vi "convertVideo.vi"(8 "error in (no error)":errorcluster, 9 "format":string, 10 "fileName":string, 11 "VideoConversionFacade in":refnum<class "VideoConversionFacade.lvclass">) -> (0 "error out":errorcluster, 2 "result out":refnum<class "VideoFile.lvclass">, 3 "VideoConversionFacade out":refnum<class "VideoConversionFacade.lvclass">)   [LabVIEW 2017, in "VideoConversionFacade.lvclass"]
uses:
  VideoConversionFacade.lvclass
  VideoFile Class/VideoFile.lvclass
  CodecFactory Class/CodecFactory.lvclass
  BitrateReader Class/BitrateReader.lvclass
  AudioMixer Class/AudioMixer.lvclass
  ConsoleOut/Print Options.ctl
  OggCompressionCodec Class/OggCompressionCodec.lvclass
  C:/Users/fflores/Documents/LabVIEW-Open-Projects/LabIVEW OOP Design Patterns/Facade Pattern/Codec Class/Codec.lvclass
  MPEG4CompressionCodec Class/MPEG4CompressionCodec.lvclass
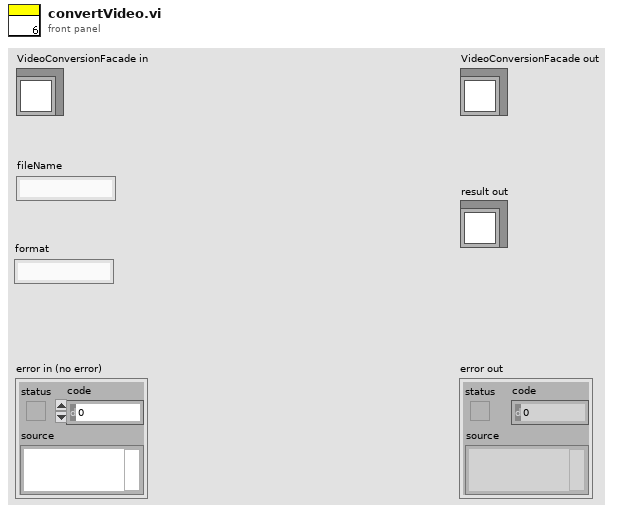
[diagram p1: front panel]
types:
  T1 = typedef "Print Options.ctl" = enum16{"Create", "Get Reference", "Print", "Print Header", "Close"}
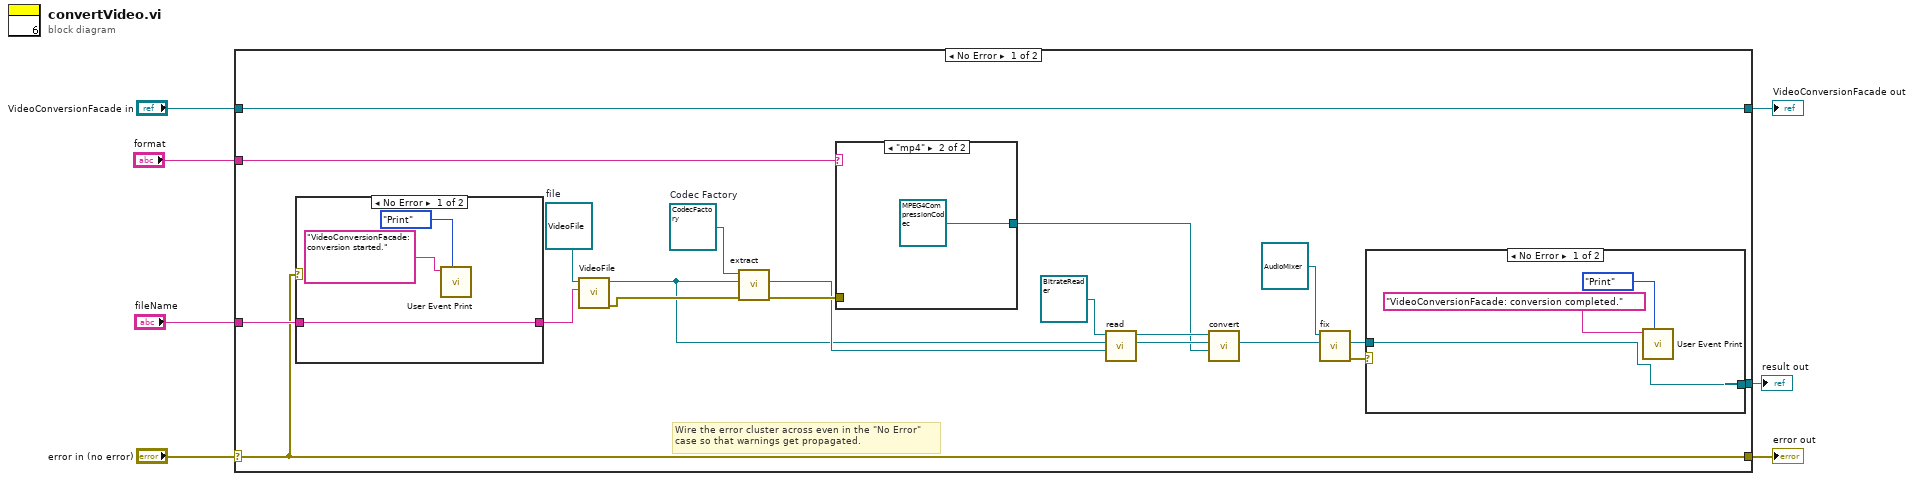
[diagram p0: block diagram]
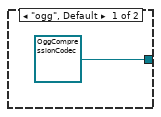
[diagram p4: hidden frame]
diagram:
  n1 = case shown="No Error" "error in (no error)" {
    selector: "error in (no error)" -> [w10 w38]
    tunnel: [w10 w38] -> w6
    tunnel: [w27 w37] -> w4
    tunnel: "VideoConversionFacade in" -> [w27 w37]
    tunnel: "fileName" -> [w12 _]
    tunnel: "format" -> [w22 _]
    tunnel: [w9 _] -> w1
    frame No Error {
      w25 = refnum<class "CodecFactory.lvclass"> refnum  # Codec Factory
      w26 = refnum<class "VideoFile.lvclass"> refnum  # file
      # "Wire the error cluster across even in the \"No Error\"\ncase so that warnings get propagated."
      n2 = case shown="No Error" w10 {
        tunnel: w12 -> [w30 w31]
        tunnel: [w30 w31] -> w11
        frame No Error {
          n3 = call "User Event Print.vi"("Options"=Print_Options."Print", "String to Print"="VideoConversionFacade: conversion started." ("message")) -> ()  [unwired: 8 in, 2 out]
        }
        frame Error {
        }
      }
      n4 = call "VideoFile.vi"("name"=w11, "VideoFile in"=w26) -> ("error out"=w24:errorcluster, "VideoFile out"=w20:refnum<class "VideoFile.lvclass">)  [unwired: 8 in]
      n5 = call "extract.vi"("error in (no error)"=w24, "VideoFile"=w20, "CodecFactory in"=w25) -> ("error out"=w23:errorcluster, "Codec"=w21:refnum<class "Codec.lvclass">)  [unwired: 6 in, 1 out]
      n6 = case shown="\"mp4\"" w22 {
        tunnel: w23 -> [_ _]
        tunnel: [refnum<class "OggCompressionCodec.lvclass"> refnum ("OggCompressionCodec.lvclass") refnum<class "MPEG4CompressionCodec.lvclass"> refnum ("MPEG4CompressionCodec.lvclass")] -> w16
        frame "ogg", Default {
        }
        frame "mp4" {
        }
      }
      n7 = call "read.vi"("Codec"=w21, "file"=w20, "BitrateReader in"=refnum<class "BitrateReader.lvclass"> refnum ("BitrateReader.lvclass")) -> ("VideoFile Out"=w17:refnum<class "VideoFile.lvclass">, "BitrateReader out"=w18:refnum<class "BitrateReader.lvclass">)  [unwired: 6 in, 1 out]
      n8 = call "convert.vi"("Codec"=w16, "buffer"=w17, "BitrateReader in"=w18) -> ("buffer out"=w15:refnum<class "VideoFile.lvclass">)  [unwired: 6 in, 2 out]
      n9 = call "fix.vi"("result"=w15, "AudioMixer in"=refnum<class "AudioMixer.lvclass"> refnum ("AudioMixer.lvclass")) -> ("error out"=w13:errorcluster, "result out"=w8:refnum<class "VideoFile.lvclass">)  [unwired: 7 in, 1 out]
      n10 = case shown="No Error" w13 {
        tunnel: [w34 _] -> w9
        tunnel: w8 -> [w34 _]
        frame No Error {
          n11 = call "User Event Print.vi"("Options"=Print_Options."Print", "String to Print"="VideoConversionFacade: conversion completed." ("message")) -> ()  [unwired: 8 in, 2 out]
        }
        frame Error {
        }
      }
    }
    frame Error {
    }
  }
  "error out" <- w6
  "VideoConversionFacade out" <- w4
  "result out" <- w1
